vi "CalculateCycleCyclePkRMS(1 CH).vi"(8 "error in (no error)":errorcluster, 10 "line frequency":dbl, 11 "waveform":waveform(dbl)) -> (0 "error out":errorcluster, 2 "peak waveform":waveform(dbl), 3 "rms waveform":waveform(dbl))   [LabVIEW 2017, in "McsaAnalysisFunctions.lvlib"]
uses:
  <vilib>/addons/InsightCM/Utilities/Analysis/MCSA/McsaAnalysisFunctions.lvlib
  <vilib>/Analysis/5stat.llb/RMS (DBL).vi
  <vilib>/Waveform/WDTOps.llb/WDT Waveform Duration DBL.vi
  <vilib>/Analysis/NI_AALPro.lvlib
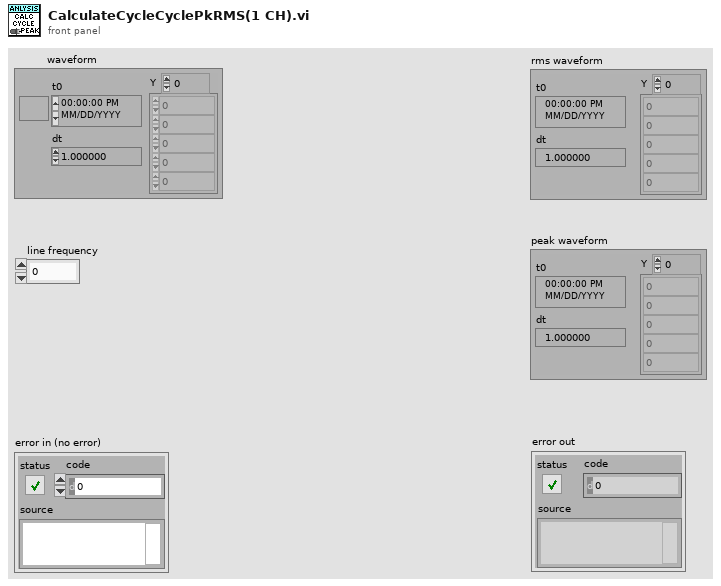
[diagram p1: front panel]
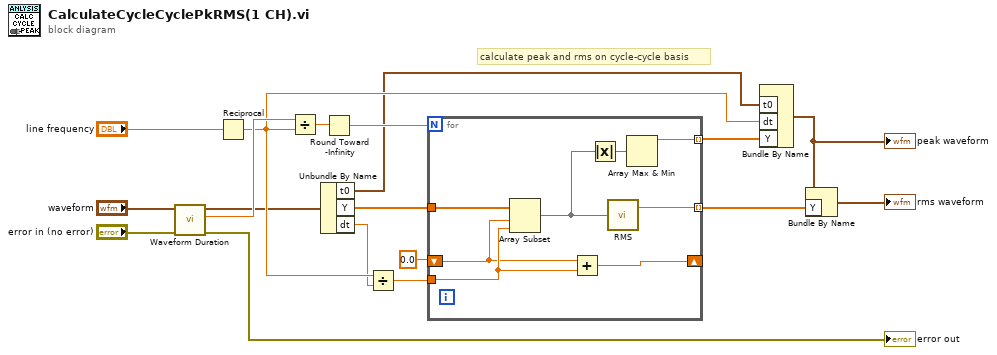
[diagram p0: block diagram]
diagram:
  # "calculate peak and rms on cycle-cycle basis"
  n1 = call-poly <vilib>:"Waveform Duration.vi"("error in (no error)"="error in (no error)", "waveform in"="waveform") -> ("error out"=→"error out":errorcluster, "duration"=w17:dbl, "waveform out"=w1:waveform(dbl))  [unwired: 7 in]
  n2 = Reciprocal(x="line frequency") -> (1/x=w7:dbl)
  n3 = Divide(x=w17, y=w7) -> (x/y=w16:dbl)
  n4 = Unbundle By Name(w1) -> ("t0"=w3:timestamp, "Y"=w8:dbl[], "dt"=w6:dbl)
  n5 = Round Toward -Infinity(1:w16) -> (0:w15:dbl)
  n6 = Divide(x=w7, y=w6) -> (x/y=w5:dbl)
  n7 = for {
    N: w15 -> [_]
    tunnel: w5 -> [w26]
    shift-right: [w24] -> _
    shift-left: 0.0 -> [w25]
    tunnel: [w22] -> w13 mode=indexing
    tunnel: [w20] -> w11 mode=indexing
    tunnel: w8 -> [w19]
    n8 = Array Subset(array=w19, index=w25, length=w26) -> (w21:dbl[])
    n9 = Add(x=w25, y=w26) -> (x+y=w24:dbl)
    n10 = Absolute Value(x=w21) -> (abs(x)=w23:dbl[])
    n11 = call-poly <vilib>:"RMS.vi"("X"=w21) -> ("rms value"=w20:dbl)  [unwired: 1 out]
    n12 = Array Max & Min(array=w23) -> (max value=w22:dbl)  [unwired: 3 out]
  }
  n13 = Bundle By Name("t0"=w3, "dt"=w7, "Y"=w13) -> (w12:waveform(dbl))  [unwired: 1 in]
  "peak waveform" <- w12
  n14 = Bundle By Name(cluster=w12, "Y"=w11) -> (→"rms waveform":waveform(dbl))
